vi "waveformparams.vi"(1 "Params in":T1, 2 "command":string="clear") -> (0 "Params out":T1)   [LabVIEW 2015]
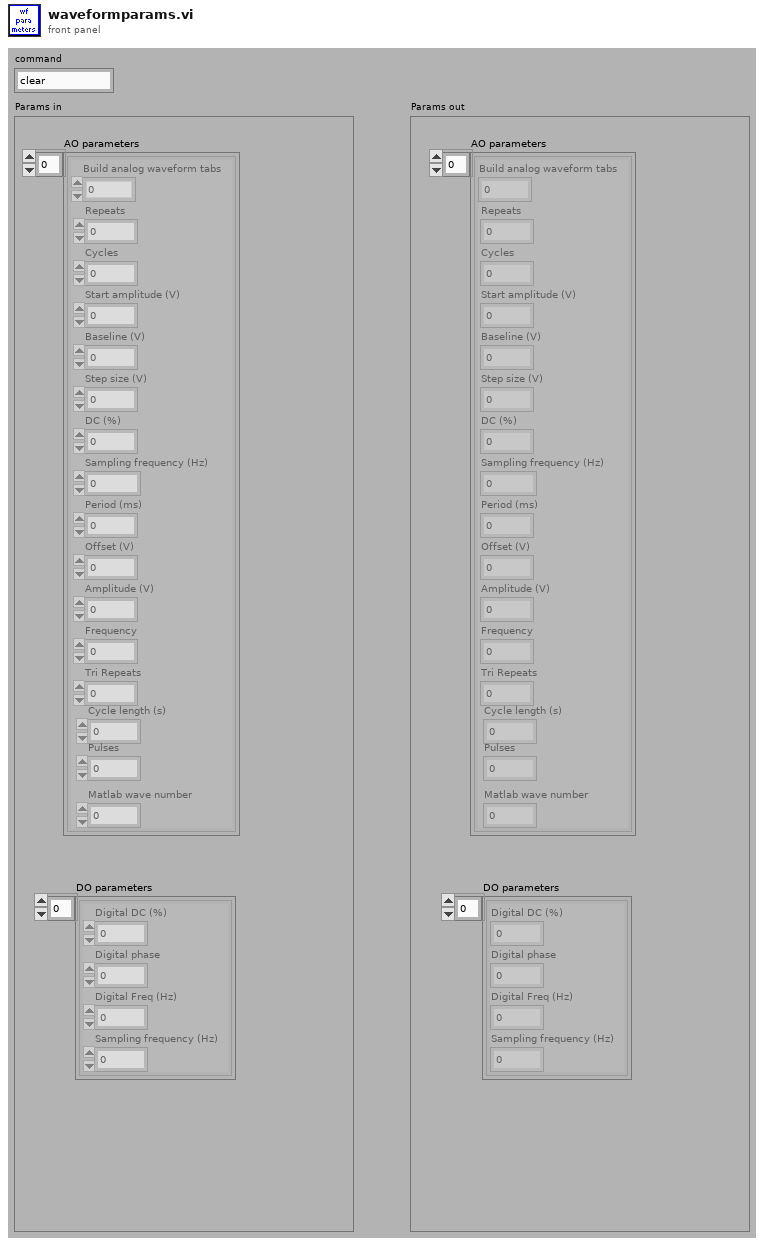
[diagram p1: front panel]
types:
  T1 = cluster{"AO parameters":cluster{"Build analog waveform tabs":dbl, "Repeats":dbl, "Cycles":dbl, "Start amplitude (V)":dbl, "Baseline (V)":dbl, "Step size (V)":dbl, "DC (%)":dbl, "Sampling frequency (Hz)":dbl, "Period (ms)":dbl, "Offset (V)":dbl, "Amplitude (V)":dbl, "Frequency":dbl, "Tri Repeats":dbl, "Cycle length (s)":dbl, "Pulses":dbl, "Matlab wave number":dbl}[], "DO parameters":cluster{"Digital DC (%)":dbl, "Digital phase":dbl, "Digital Freq (Hz)":dbl, "Sampling frequency (Hz)":dbl}[]}
  T2 = cluster{"Digital DC (%)":dbl, "Digital phase":dbl, "Digital Freq (Hz)":dbl, "Sampling frequency (Hz)":dbl}[]
  T3 = cluster{"Build analog waveform tabs":dbl, "Repeats":dbl, "Cycles":dbl, "Start amplitude (V)":dbl, "Baseline (V)":dbl, "Step size (V)":dbl, "DC (%)":dbl, "Sampling frequency (Hz)":dbl, "Period (ms)":dbl, "Offset (V)":dbl, "Amplitude (V)":dbl, "Frequency":dbl, "Tri Repeats":dbl, "Cycle length (s)":dbl, "Pulses":dbl, "Matlab wave number":dbl}[]
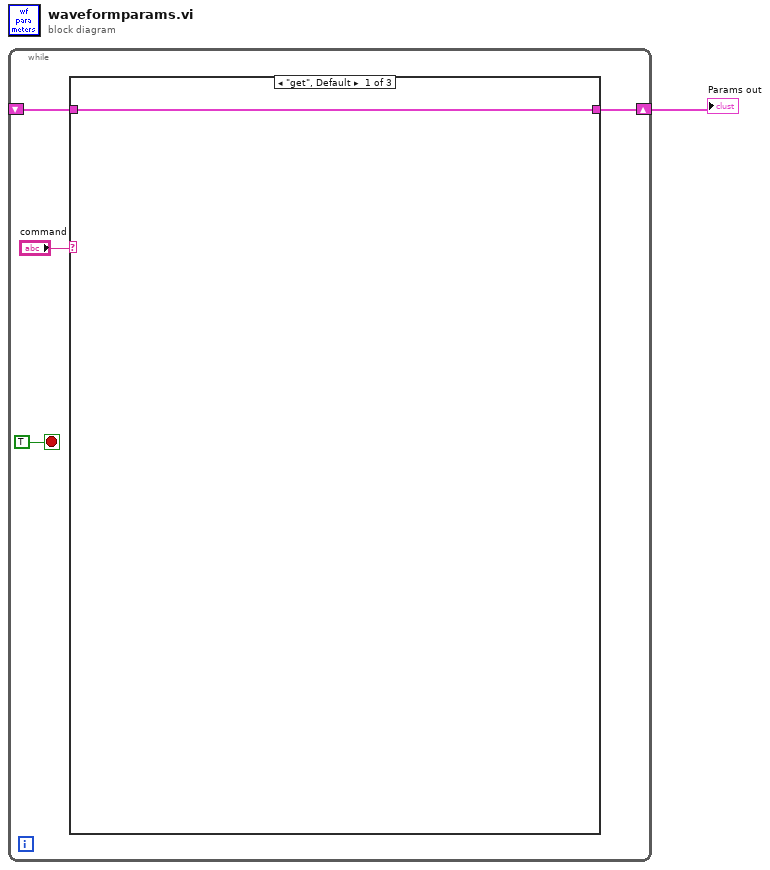
[diagram p0: block diagram]
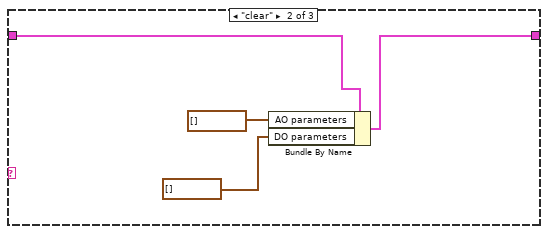
[diagram p2: hidden frame]
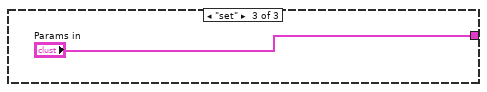
[diagram p3: hidden frame]
diagram:
  n1 = while {
    shift-right: [w3] -> w1
    shift-left: _ -> [w2]
    stop <- TRUE stop-if-true
    n2 = case shown="\"get\", Default" "command" {
      tunnel: [w6 w9 "Params in"] -> w3
      tunnel: w2 -> [w6 w10 _]
      frame "get", Default {
      }
      frame "clear" {
        n3 = Bundle By Name(cluster=w10, "AO parameters"=T3 [], "DO parameters"=T2 []) -> (w9:T1)
      }
      frame "set" {
      }
    }
  }
  "Params out" <- w1
